vi "Set Gear Ratio.vi"(8 "error in (no error)":errorcluster, 10 "gear ratio":dbl, 11 "wheel in":refnum<class "NI_Robotics_Wheel.lvclass">) -> (0 "error out":errorcluster, 3 "wheel out":refnum<class "NI_Robotics_Wheel.lvclass">)   [LabVIEW 2017, in "NI_Robotics_Wheel.lvclass"]
uses:
  <vilib>/robotics/Steering/Wheel/NI_Robotics_Wheel.lvclass
  <vilib>/robotics/Steering/Wheel/NI_Robotics_Wheel.lvclass/NI_Robotics_Wheel.ctl
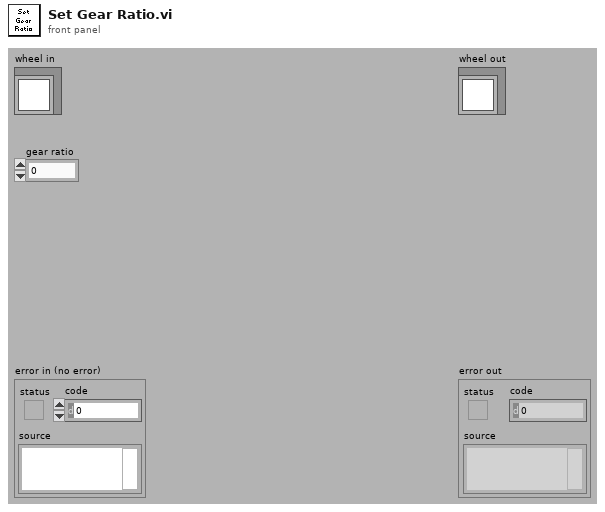
[diagram p1: front panel]
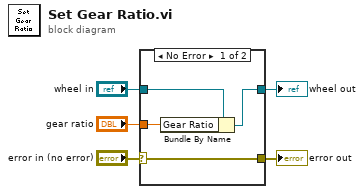
[diagram p0: block diagram]
diagram:
  n1 = case shown="No Error" "error in (no error)" {
    selector: "error in (no error)" -> [w9 w11]
    tunnel: [w9 w11] -> w4
    tunnel: [w6 w10] -> w2
    tunnel: "wheel in" -> [w7 w10]
    tunnel: "gear ratio" -> [w8 _]
    frame No Error {
      n2 = Bundle By Name(cluster=w7, "Gear Ratio"=w8) -> (w6:refnum<class "NI_Robotics_Wheel.lvclass">)
    }
    frame Error {
    }
  }
  "error out" <- w4
  "wheel out" <- w2
